vi "Inject.vi"(10 "NumToInject":i32, 11 "Array In":dbl[][](array[numeric])) -> (3 "Array Out":dbl[][](array[numeric]))   [LabVIEW 2016]
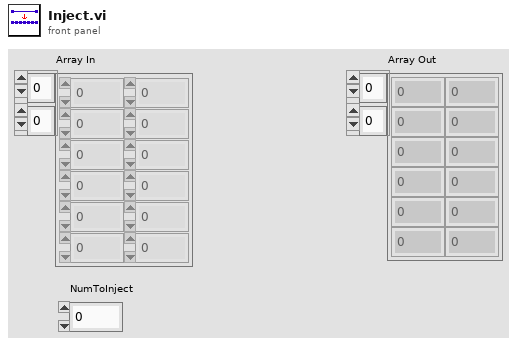
[diagram p1: front panel]
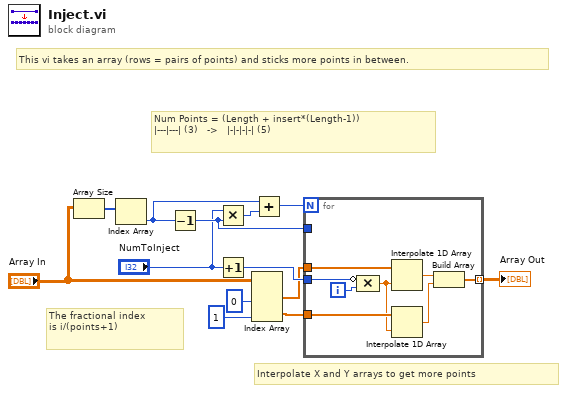
[diagram p0: block diagram]
diagram:
  # "The fractional index\nis i/(points+1)"
  # "Interpolate X and Y arrays to get more points"
  # "This vi takes an array (rows = pairs of points) and sticks more points in between."
  # "Num Points = (Length + insert*(Length-1))\n|---|---| (3)   ->   |-|-|-|-| (5)"
  n1 = Array Size(array="Array In") -> (size(s)=w13:i32[])
  n2 = Index Array(array=w13) -> (element=w10:i32)  [unwired: 1 in]
  n3 = Decrement(x=w10) -> (x-1=w9:i32)
  n4 = Multiply(x="NumToInject", y=w9) -> (x*y=w12:i32)
  n5 = Increment(x="NumToInject") -> (x+1=w7:i32)
  n6 = Index Array(array="Array In", index (col) #1=0 ("disabled index (col)"), index (col) #2=1 ("index (col)")) -> (element #1=w2:dbl[], element #2=w1:dbl[])  [unwired: 2 in]
  n7 = Add(x=w10, y=w12) -> (x+y=w11:i32)
  n8 = for {
    N: w11 -> [_]
    tunnel: w2 -> [w20]
    tunnel: w1 -> [w18]
    tunnel: w9 -> [_]
    tunnel: w7 -> [w19]
    tunnel: [w14] -> w6 mode=indexing
    i -> [w21]
    n9 = Compound Arithmetic op=MULTIPLY(invert w19, w21) -> (w17:dbl)
    n10 = Interpolate 1D Array(1:w17, 2:w20) -> (0:w16:dbl)
    n11 = Interpolate 1D Array(1:w17, 2:w18) -> (0:w15:dbl)
    n12 = Build Array(w16, w15) -> (w14:dbl[])
  }
  "Array Out" <- w6
